vi "Run.vi"(8 "error in (no error)":errorcluster, 9 "s on last turn":dbl, 10 "Maze (0: Empty, -1: Enemy. >0: Teammate":i32[][](array[numeric]), 11 "Expand in":refnum<class "Cautious Wolf.lvclass">) -> (0 "error out":errorcluster, 1 "Direction":T1, 2 "Action":T2, 3 "Expand out":refnum<class "Cautious Wolf.lvclass">, 4 "Replicated":refnum<class "Square.lvclass">)   [LabVIEW 2015, in "Cautious Wolf.lvclass"]
uses:
  Cautious Wolf.lvclass
  Type Defs/Action Enum.ctl
  Type Defs/Direction Enum.ctl
  Square/Square.lvclass
  Cautious Wolf.lvclass/Cautious Wolf.ctl
  SubVIs/Read-Only Globals.vi
  Type Defs/SB Type Defs.lvlib
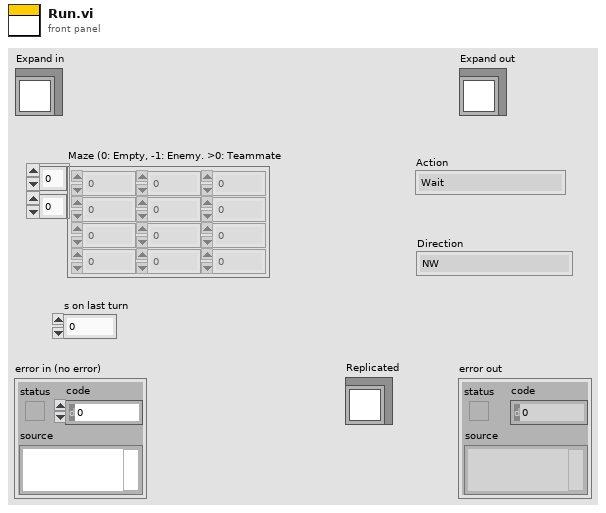
[diagram p1: front panel]
types:
  T1 = typedef "SB Type Defs.lvlib/Direction Enum.ctl" = enum16{"NW", "N", "NE", "E", "SE", "S", "SW", "W"}
  T2 = typedef "SB Type Defs.lvlib/Action Enum.ctl" = enum16{"Wait", "Move", "Attack", "Replicate"}
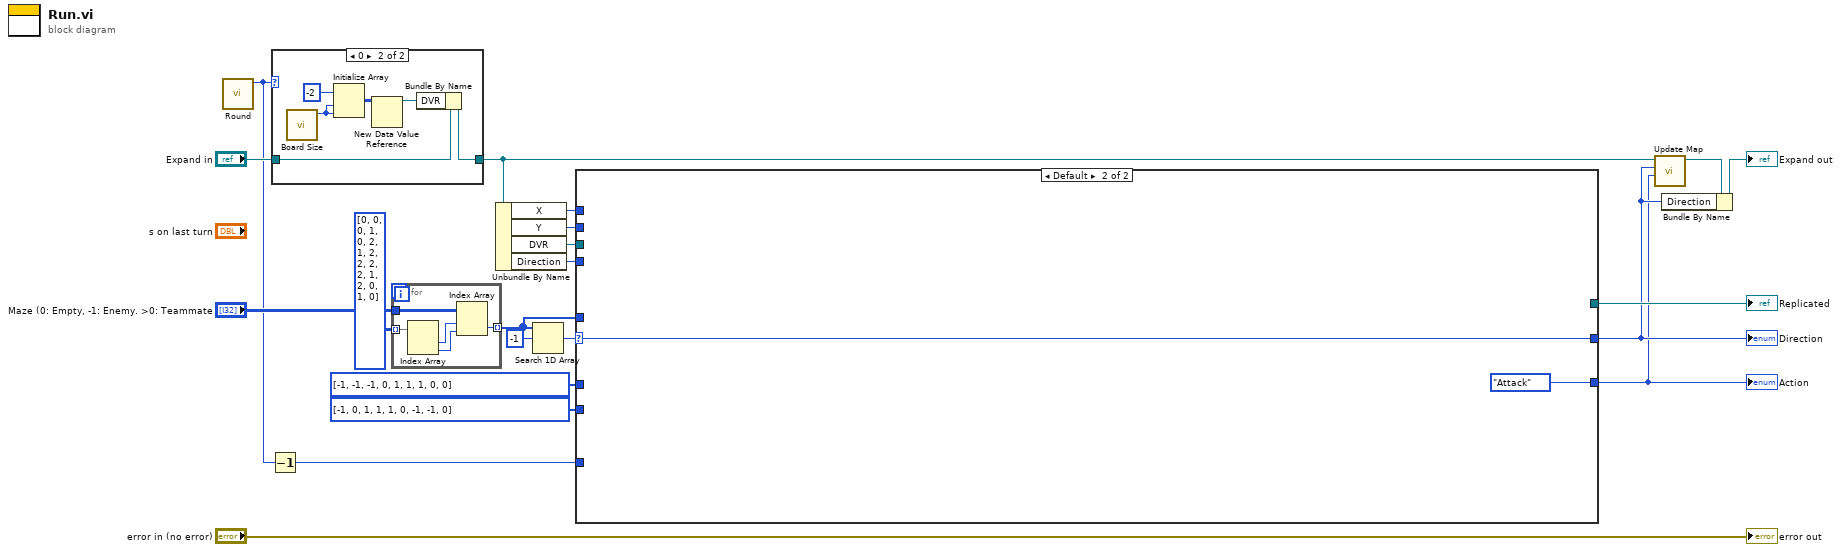
[diagram p0: block diagram]
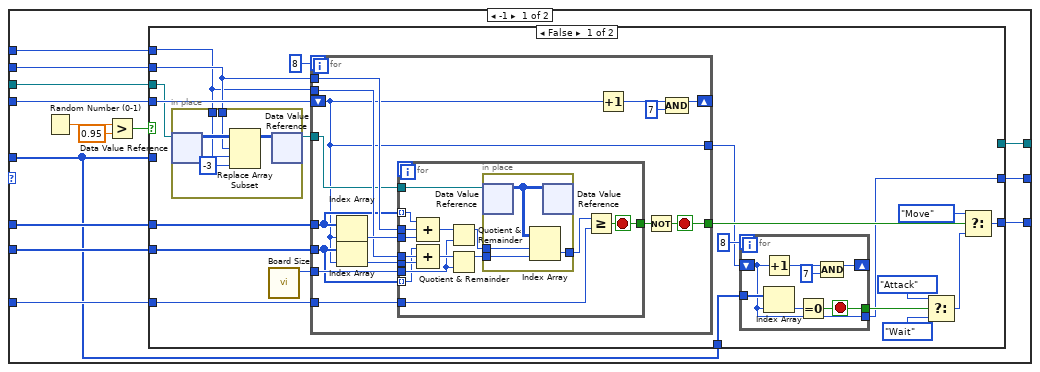
[diagram p3: hidden frame]
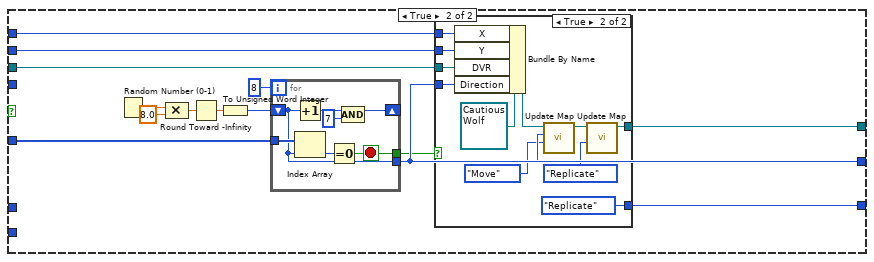
[diagram p4: hidden frame]
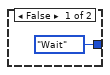
[diagram p5: hidden frame]
diagram:
  n1 = call "Round.vi"() -> ("Round"=w2:i32)  [unwired: 11 in]
  n2 = Decrement(x=w2) -> (x-1=w1:i32)
  n3 = case shown="0" w2 {
    tunnel: "Expand in" -> [w22 w26]
    tunnel: [w22 w24] -> w9
    frame Default {
    }
    frame 0 {
      n4 = call "Board Size.vi"() -> ("Board Size"=w23:i32)  [unwired: 11 in]
      n5 = Initialize Array(-2, w23, w23) -> (w27:i32[][])
      n6 = New Data Value Reference(data value=w27) -> (data value reference=w25:refnum<data-value>)  [unwired: 1 in, 1 out]
      n7 = Bundle By Name(cluster=w26, "DVR"=w25) -> (w24:refnum<class "Cautious Wolf.lvclass">)
    }
  }
  n8 = for {
    tunnel: "Maze (0: Empty, -1: Enemy. >0: Teammate" -> [w33]
    tunnel: i32[][] [[0, 0], [0, 1], [0, 2], [1, 2], [2, 2], [2, 1], [2, 0], [1, 0]] -> [w32] mode=indexing
    tunnel: [w29] -> w16 mode=indexing
    n9 = Index Array(array=w32) -> (element #1=w31:i32, element #2=w30:i32)  [unwired: 2 in]
    n10 = Index Array(array=w33, index (row)=w31, index (col)=w30) -> (element=w29:i32)
  }
  n11 = Unbundle By Name(w9) -> ("X"=w5:i32, "Y"=w6:i32, "DVR"=w11:refnum<data-value>, "Direction"=w13:T1)
  n12 = Search 1D Array(1D array=w16, element=-1) -> (index of element=w17:i32)  [unwired: 1 in]
  n13 = case shown="Default" w17 {
    selector: w17 -> [_ w148]
    tunnel: [w43 w148] -> w8
    tunnel: [w47 Action_Enum."Attack" ("Action")] -> w7
    tunnel: w16 -> [w34 _]
    tunnel: [w46 _] -> w15
    tunnel: w13 -> [w38 _]
    tunnel: w11 -> [w41 _]
    tunnel: w6 -> [w40 _]
    tunnel: w5 -> [w39 _]
    tunnel: i32[] [-1, -1, -1, 0, 1, 1, 1, 0, 0] -> [w37 _]
    tunnel: i32[] [-1, 0, 1, 1, 1, 0, -1, -1, 0] -> [w36 _]
    tunnel: w1 -> [w35 _]
    frame -1 {
      n14 = Random Number (0-1)() -> (number: 0 to 1=w44:dbl)
      n15 = Greater?(x=w44, y=0.95) -> (0:w42:bool)
      n16 = case shown="False" w42 {
        tunnel: [w56 w128] -> w47
        tunnel: [_ w116] -> w46
        tunnel: w34 -> [_ w126]
        tunnel: [w48 w117] -> w43
        tunnel: w41 -> [w63 w120]
        tunnel: w40 -> [w62 w119]
        tunnel: w39 -> [w61 w118]
        tunnel: w38 -> [w67 _]
        tunnel: w37 -> [w65 _]
        tunnel: w36 -> [w66 _]
        tunnel: w35 -> [w59 _]
        tunnel: w34 -> [w54 _]
        frame False {
          n17 = in-place {
            in-place-border: w62 -> [w78]
            in-place-border: w61 -> [w77]
            n18 = in-place-dvr #1(w63) -> (w80:i32[][])  [unwired: 1 out]
            n19 = Replace Array Subset(array=w80, new element=-3 ("new element/subarray"), index (row)=w78, index (col)=w77) -> (w79:i32[][])
            n20 = in-place-dvr #1(w79) -> (w60:refnum<data-value>)  [unwired: 1 out]
          }
          n21 = call "Board Size.vi"() -> ("Board Size"=w64:i32)  [unwired: 11 in]
          n22 = for {
            N: 8 -> [_]
            shift-right: [w93] -> _
            shift-left: w67 -> [w81]
            tunnel: w66 -> [w86]
            tunnel: w65 -> [w87]
            tunnel: w64 -> [w90]
            tunnel: w62 -> [w89]
            tunnel: w61 -> [w88]
            tunnel: w60 -> [w84]
            tunnel: w59 -> [w85]
            tunnel: [w82] -> w58
            tunnel: [w81] -> w53
            stop <- w82 stop-if-true
            n23 = Index Array(array=w87, index=w81) -> (element=w92:i32)
            n24 = Index Array(array=w86, index=w81) -> (element=w91:i32)
            n25 = for {
              tunnel: w92 -> [w108]
              tunnel: w91 -> [w107]
              tunnel: w90 -> [w106]
              tunnel: w89 -> [w105]
              tunnel: w88 -> [w104]
              tunnel: w87 -> [w103] mode=indexing
              tunnel: w86 -> [w102] mode=indexing
              tunnel: w85 -> [w97]
              tunnel: w84 -> [w101]
              tunnel: [w96] -> w83
              stop <- w96 stop-if-true
              n26 = Compound Arithmetic op=ADD(w103, w105, w108) -> (w109:i32)
              n27 = Compound Arithmetic op=ADD(w102, w104, w107) -> (w110:i32)
              n28 = Quotient & Remainder(x=w109, y=w106) -> (x-y*floor(x/y)=w100:i32)  [unwired: 1 out]
              n29 = Quotient & Remainder(x=w110, y=w106) -> (x-y*floor(x/y)=w99:i32)  [unwired: 1 out]
              n30 = in-place {
                in-place-border: w100 -> [w113]
                in-place-border: w99 -> [w112]
                in-place-border: [w111] -> w98
                n31 = in-place-dvr #2(w101) -> (w114:i32[][])  [unwired: 1 out]
                n32 = Index Array(array=w114, index (row)=w113, index (col)=w112) -> (element=w111:i32)
                n33 = in-place-dvr #2(w114) -> ()  [unwired: 2 out]
              }
              n34 = Greater Or Equal?(x=w98, y=w97) -> (x >= y?=w96:bool)
            }
            n35 = Increment(x=w81) -> (x+1=w95:i32)
            n36 = Not(x=w83) -> (.not. x?=w82:bool)
            n37 = Compound Arithmetic op=AND(w95, 7) -> (w93:i32)
          }
          n38 = for {
            N: 8 -> [_]
            tunnel: w54 -> [w75]
            shift-right: [w69] -> _
            shift-left: w53 -> [w73]
            tunnel: [w73] -> w48
            tunnel: [w72] -> w52
            stop <- w72 stop-if-true
            n39 = Increment(x=w73) -> (x+1=w70:i32)
            n40 = Index Array(array=w75, index=w73) -> (element=w74:i32)
            n41 = Equal To 0?(x=w74) -> (x = 0?=w72:bool)
            n42 = Compound Arithmetic op=AND(w70, 7) -> (w69:i32)
          }
          n43 = Select(t=Action_Enum."Attack" ("y"), s=w52, f=Action_Enum."Wait" ("y")) -> (s? t:f=w50:T2)
          n44 = Select(t=Action_Enum."Move" ("y"), s=w58, f=w50) -> (s? t:f=w56:T2)
        }
        frame True {
          n45 = Random Number (0-1)() -> (number: 0 to 1=w122:dbl)
          n46 = Compound Arithmetic op=MULTIPLY(w122, 8.0 ("value")) -> (w124:dbl)
          n47 = Round Toward -Infinity(1:w124) -> (0:w125:dbl)
          n48 = To Unsigned Word Integer(number=w125) -> (unsigned 16bit integer=w121:u16)
          n49 = for {
            N: 8 -> [_]
            tunnel: w126 -> [w147]
            shift-right: [w141] -> _
            shift-left: w121 -> [w145]
            tunnel: [w145] -> w117
            tunnel: [w144] -> w115
            stop <- w144 stop-if-true
            n50 = Increment(x=w145) -> (x+1=w142:u16)
            n51 = Index Array(array=w147, index=w145) -> (element=w146:i32)
            n52 = Equal To 0?(x=w146) -> (x = 0?=w144:bool)
            n53 = Compound Arithmetic op=AND(w142, u16 7 ("x+1")) -> (w141:u16)
          }
          n54 = case shown="True" w115 {
            tunnel: [Action_Enum."Wait" ("y") Action_Enum."Replicate" ("y")] -> w128
            tunnel: w120 -> [_ w138]
            tunnel: w119 -> [_ w137]
            tunnel: w118 -> [_ w136]
            tunnel: w117 -> [_ w134]
            tunnel: [_ w131] -> w116
            frame False {
            }
            frame True {
              n55 = Bundle By Name(cluster=refnum<class "Cautious Wolf.lvclass"> refnum ("Lone Wolf.lvclass"), "X"=w136, "Y"=w137, "DVR"=w138, "Direction"=w134) -> (w135:refnum<class "Cautious Wolf.lvclass">)
              n56 = call "Update Map.vi"("Action"=Action_Enum."Move", "Direction"=w134, "Class"=w135) -> ("Class"=w132:refnum<class "Cautious Wolf.lvclass">)  [unwired: 8 in]
              n57 = call "Update Map.vi"("Action"=Action_Enum."Replicate", "Class"=w132) -> ("Class"=w131:refnum<class "Cautious Wolf.lvclass">)  [unwired: 9 in]
            }
          }
        }
      }
    }
    frame Default {
    }
  }
  "Action" <- w7
  "Direction" <- w8
  "Replicated" <- w15
  n58 = call "Update Map.vi"("Action"=w7, "Direction"=w8, "Class"=w9) -> ("Class"=w10:refnum<class "Cautious Wolf.lvclass">)  [unwired: 8 in]
  n59 = Bundle By Name(cluster=w10, "Direction"=w8) -> (→"Expand out":refnum<class "Cautious Wolf.lvclass">)
  "error out" <- "error in (no error)"
